vi "Read Data and Draw to LV Picture.vi"(6 "Pixel Format":string, 8 "error in (no error)":errorcluster, 11 "Buffer in":refnum<class "Buffer.lvclass">) -> (0 "error out":errorcluster, 2 "Picture":picture, 3 "Buffer out":refnum<class "Buffer.lvclass">)   [LabVIEW 2020]
uses:
  g_industrial_cam/Buffer/Buffer.lvclass
  g_industrial_cam/Buffer/Buffer.lvclass/Buffer.ctl
  g_industrial_cam/Buffer/Read Data as Mono8 Image.vi
  g_industrial_cam/Buffer/Read Data as Mono10 Image.vi
  g_industrial_cam/Buffer/Read Data as Mono10p Image.vi
  g_industrial_cam/Buffer/Read Data as Mono12 Image.vi
  g_industrial_cam/Buffer/Read Data as Mono12p Image.vi
  g_industrial_cam/Buffer/Read Data as Mono14 Image.vi
  g_industrial_cam/Buffer/Read Data as Mono14p Image.vi
  g_industrial_cam/Buffer/Read Data as Mono16 Image.vi
  g_industrial_cam/Buffer/Draw RGB8 to Picture.vi
  g_industrial_cam/Buffer/ReadDataAsMono2Byte.vi
  g_industrial_cam/Buffer/DrawToPictureCore.vi
  <vilib>/picture/picture.llb/Draw 8-Bit Pixmap.vi
  g_industrial_cam/Buffer/Draw BGR8 to Picture.vi
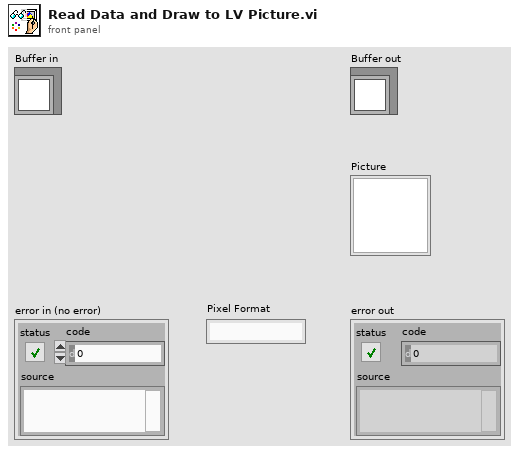
[diagram p1: front panel]
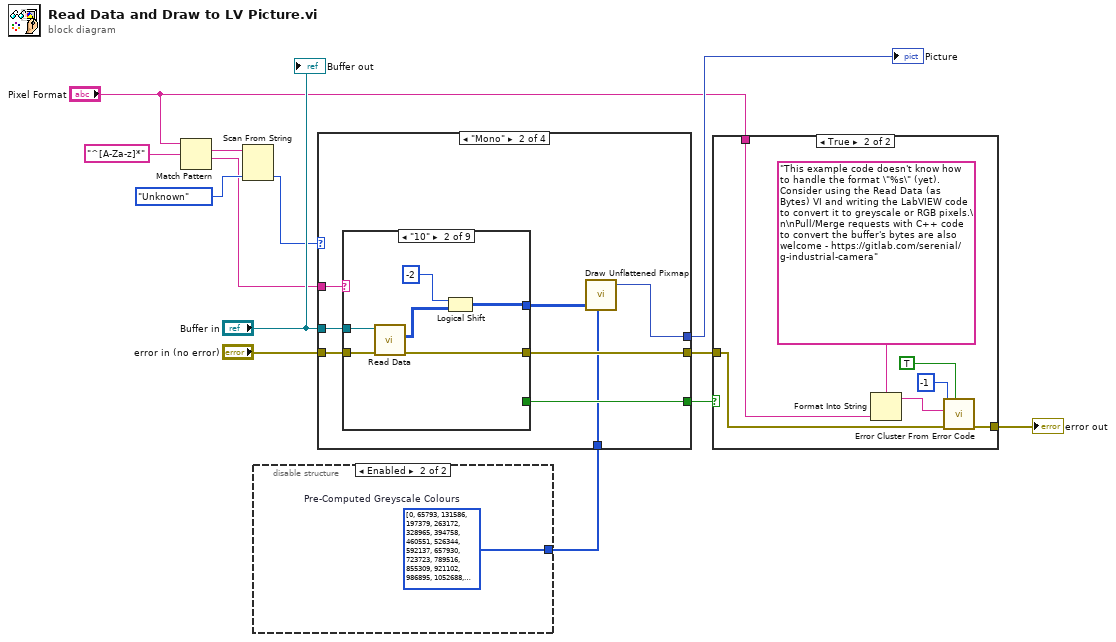
[diagram p0: block diagram]
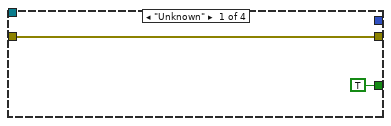
[diagram p3: hidden frame]
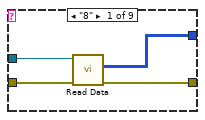
[diagram p4: hidden frame]
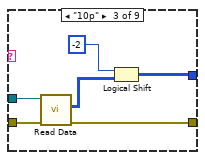
[diagram p5: hidden frame]
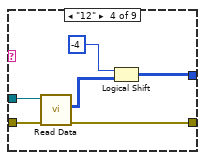
[diagram p6: hidden frame]
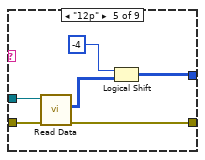
[diagram p7: hidden frame]
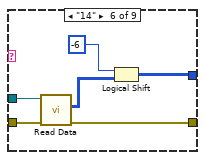
[diagram p8: hidden frame]
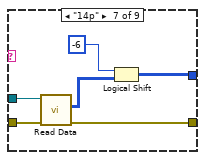
[diagram p9: hidden frame]
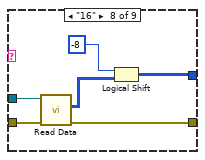
[diagram p10: hidden frame]
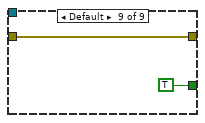
[diagram p11: hidden frame]
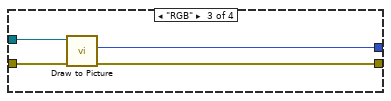
[diagram p12: hidden frame]
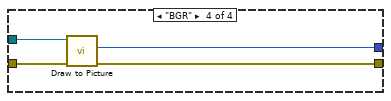
[diagram p13: hidden frame]
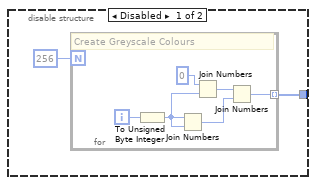
[diagram p14: hidden frame]
diagram:
  n1 = Match Pattern(string="Pixel Format", regular expression="^[A-Za-z]*") -> (match substring=w10:string, after substring=w7:string)  [unwired: 1 in, 2 out]
  n2 = Scan From String(input string=w10, default 1=enum16{"Unknown", "Mono", "RGB", "BGR"}."Unknown") -> (output 1=w8:enum16{"Unknown", "Mono", "RGB", "BGR"})  [unwired: 3 in, 3 out]
  n3 = disable-structure shown="Enabled" {
    disable-tunnel: [w14 w22] -> w1
    frame Disabled {
      n4 = for {
        N: 256 -> [_]
        tunnel: [w16] -> w14 mode=indexing
        i -> [w21]
        # "Create Greyscale Colours"
        n5 = To Unsigned Byte Integer(number=w21) -> (unsigned 8bit integer=w20:u8)
        n6 = Join Numbers(hi=w20, lo=w20) -> ((hi.lo)=w17:u16)
        n7 = Join Numbers(hi=u8 0, lo=w20) -> ((hi.lo)=w18:u16)
        n8 = Join Numbers(hi=w18, lo=w17) -> ((hi.lo)=w16:u32)
      }
    }
    frame Enabled {
      w22 = u32[] [0, 65793, 131586, 197379, 263172, 328965, 394758, 460551, 526344, 592137, 657930, 723723, 789516, 855309, 921102, 986895, 1052688, 1118481, 1184274, 1250067, 1315860, 1381653, 1447446, 1513239, 1579032, 1644825, 1710618, 1776411, 1842204, 1907997, 1973790, 2039583, 2105376, 2171169, 2236962, 2302755, 2368548, 2434341, 2500134, 2565927, 2631720, 2697513, 2763306, 2829099, 2894892, 2960685, 3026478, 3092271, 3158064, 3223857, 3289650, 3355443, 3421236, 3487029, 3552822, 3618615, 3684408, 3750201, 3815994, 3881787, 3947580, 4013373, 4079166, 4144959, 4210752, 4276545, 4342338, 4408131, 4473924, 4539717, 4605510, 4671303, 4737096, 4802889, 4868682, 4934475, 5000268, 5066061, 5131854, 5197647, 5263440, 5329233, 5395026, 5460819, 5526612, 5592405, 5658198, 5723991, 5789784, 5855577, 5921370, 5987163, 6052956, 6118749, 6184542, 6250335, 6316128, 6381921, 6447714, 6513507, 6579300, 6645093, 6710886, 6776679, 6842472, 6908265, 6974058, 7039851, 7105644, 7171437, 7237230, 7303023, 7368816, 7434609, 7500402, 7566195, 7631988, 7697781, 7763574, 7829367, 7895160, 7960953, 8026746, 8092539, 8158332, 8224125, 8289918, 8355711, 8421504, 8487297, 8553090, 8618883, 8684676, 8750469, 8816262, 8882055, 8947848, 9013641, 9079434, 9145227, 9211020, 9276813, 9342606, 9408399, 9474192, 9539985, 9605778, 9671571, 9737364, 9803157, 9868950, 9934743, 10000536, 10066329, 10132122, 10197915, 10263708, 10329501, 10395294, 10461087, 10526880, 10592673, 10658466, 10724259, 10790052, 10855845, 10921638, 10987431, 11053224, 11119017, 11184810, 11250603, 11316396, 11382189, 11447982, 11513775, 11579568, 11645361, 11711154, 11776947, 11842740, 11908533, 11974326, 12040119, 12105912, 12171705, 12237498, 12303291, 12369084, 12434877, 12500670, 12566463, 12632256, 12698049, 12763842, 12829635, 12895428, 12961221, 13027014, 13092807, 13158600, 13224393, 13290186, 13355979, 13421772, 13487565, 13553358, 13619151, 13684944, 13750737, 13816530, 13882323, 13948116, 14013909, 14079702, 14145495, 14211288, 14277081, 14342874, 14408667, 14474460, 14540253, 14606046, 14671839, 14737632, 14803425, 14869218, 14935011, 15000804, 15066597, 15132390, 15198183, 15263976, 15329769, 15395562, 15461355, 15527148, 15592941, 15658734, 15724527, 15790320, 15856113, 15921906, 15987699, 16053492, 16119285, 16185078, 16250871, 16316664, 16382457, 16448250, 16514043, 16579836, 16645629, 16711422, 16777215]  # Pre-Computed Greyscale Colours
    }
  }
  n9 = case shown="\"Mono\"" w8 {
    tunnel: "Buffer in" -> [_ w30 w83 w87]
    tunnel: "error in (no error)" -> [w23 w31 w84 w88]
    tunnel: w7 -> [_ w32 _ _]
    tunnel: [w23 w28 w82 w85] -> w4
    tunnel: [_ w27 w81 w86] -> w6
    tunnel: [TRUE w26 _ _] -> w5
    tunnel: w1 -> [_ w25 _ _]
    frame "Unknown" {
    }
    frame "Mono" {
      n10 = case shown="\"10\"" w32 {
        tunnel: w31 -> [w36 w42 w48 w54 w60 w66 w72 w78 w80]
        tunnel: w30 -> [w35 w41 w47 w53 w59 w65 w71 w77 _]
        tunnel: [w34 w38 w44 w50 w56 w62 w68 w74 _] -> w29
        tunnel: [w33 w40 w46 w52 w58 w64 w70 w76 w80] -> w28
        tunnel: [_ _ _ _ _ _ _ _ TRUE] -> w26
        frame "8" {
          n11 = call-poly "Read Data.vi"("error in (no error)"=w36, "Buffer in"=w35) -> ("error out"=w33:errorcluster, "Image"=w34:u8[][])  [unwired: 7 in, 1 out]
        }
        frame "10" {
          n12 = call-poly "Read Data.vi"("error in (no error)"=w42, "Buffer in"=w41) -> ("error out"=w40:errorcluster, "Image"=w39:u16[][])  [unwired: 7 in, 1 out]
          n13 = Logical Shift(y=i16 -2, x=w39) -> (x << y=w38:u16[][])
        }
        frame "10p" {
          n14 = call-poly "Read Data.vi"("error in (no error)"=w48, "Buffer in"=w47) -> ("error out"=w46:errorcluster, "Image"=w45:u16[][])  [unwired: 7 in, 1 out]
          n15 = Logical Shift(y=i16 -2, x=w45) -> (x << y=w44:u16[][])
        }
        frame "12" {
          n16 = call-poly "Read Data.vi"("error in (no error)"=w54, "Buffer in"=w53) -> ("error out"=w52:errorcluster, "Image"=w51:u16[][])  [unwired: 7 in, 1 out]
          n17 = Logical Shift(y=i16 -4, x=w51) -> (x << y=w50:u16[][])
        }
        frame "12p" {
          n18 = call-poly "Read Data.vi"("error in (no error)"=w60, "Buffer in"=w59) -> ("error out"=w58:errorcluster, "Image"=w57:u16[][])  [unwired: 7 in, 1 out]
          n19 = Logical Shift(y=i16 -4, x=w57) -> (x << y=w56:u16[][])
        }
        frame "14" {
          n20 = call-poly "Read Data.vi"("error in (no error)"=w66, "Buffer in"=w65) -> ("error out"=w64:errorcluster, "Image"=w63:u16[][])  [unwired: 7 in, 1 out]
          n21 = Logical Shift(y=i16 -6, x=w63) -> (x << y=w62:u16[][])
        }
        frame "14p" {
          n22 = call-poly "Read Data.vi"("error in (no error)"=w72, "Buffer in"=w71) -> ("error out"=w70:errorcluster, "Image"=w69:u16[][])  [unwired: 7 in, 1 out]
          n23 = Logical Shift(y=i16 -6, x=w69) -> (x << y=w68:u16[][])
        }
        frame "16" {
          n24 = call-poly "Read Data.vi"("error in (no error)"=w78, "Buffer in"=w77) -> ("error out"=w76:errorcluster, "Image"=w75:u16[][])  [unwired: 7 in, 1 out]
          n25 = Logical Shift(y=i16 -8, x=w75) -> (x << y=w74:u16[][])
        }
        frame Default {
        }
      }
      n26 = call-poly <vilib>:"Draw Unflattened Pixmap.vi"("data"=w29, "color table"=w25) -> ("new picture"=w27:picture)  [unwired: 7 in]
    }
    frame "RGB" {
      n27 = call-poly "Draw to Picture.vi"("error in (no error)"=w84, "Buffer in"=w83) -> ("error out"=w82:errorcluster, "Picture"=w81:picture)  [unwired: 7 in, 1 out]
    }
    frame "BGR" {
      n28 = call-poly "Draw to Picture.vi"("error in (no error)"=w88, "Buffer in"=w87) -> ("error out"=w85:errorcluster, "Picture"=w86:picture)  [unwired: 7 in, 1 out]
    }
  }
  "Picture" <- w6
  n29 = case shown="True" w5 {
    tunnel: w4 -> [w89 w92]
    tunnel: "Pixel Format" -> [_ w91]
    tunnel: [w89 w90] -> w2
    frame False {
    }
    frame True {
      n30 = Format Into String(format string="This example code doesn't know how to handle the format \"%s\" (yet). Consider using the Read Data (as Bytes) VI and writing the LabVIEW code to convert it to greyscale or RGB pixels.\n\nPull/Merge requests with C++ code to convert the buffer's bytes are also welcome - https://gitlab.com/serenial/g-industrial-camera", w91) -> (resulting string=w96:string)  [unwired: 2 in, 1 out]
      n31 = call <vilib>:"Error Cluster From Error Code.vi"("show call chain? (False)"=TRUE, "error in (no error)"=w92, "error message (\"\")"=w96, "error code (0)"=-1) -> ("error out"=w90:errorcluster)  [unwired: 5 in]
    }
  }
  "error out" <- w2
  "Buffer out" <- "Buffer in"
